vi "DataViewer.vi"() -> ()   [LabVIEW 2013]
uses:
  <vilib>/Utility/file.llb/Read From Spreadsheet File (string).vi
  <vilib>/Utility/file.llb/Read From Spreadsheet File (DBL).vi
  <vilib>/Analysis/1siggen.llb/Ramp Pattern by Delta.vi
  <vilib>/regexp/Match Regular Expression.xnode
  <vilib>/Analysis/NI_AALBase.lvlib
panel:
  in  "View Ref":bool
  out "selected reference":path caption="selected path"
  out "Polar Plot 4":picture
  out "XY Graph 3":cluster{dbl[], dbl[]}(graph)
  out "Current Freq. 2":dbl
  in  "Update 3":bool
  out "Ref In Use":bool
  in  "Remove Ref":bool
  in  "Use Reference":bool
  in  "Choose Reference Measurement":bool
  out "XY Graph 2":cluster{dbl[], dbl[]}(graph)
  in  "Update 2":bool
  out "XY Graph":cluster{dbl[], dbl[]}(graph)
  out "Current Angle":dbl
  out "Current Freq.":dbl
  in  "Update":bool
  out "Polar Plot":picture
  in  "Select Angle":dbl(slide) min=0.0 max=360.0 step=1.0 scale=0.0..360.0
  in  "Select Frequency":dbl(slide) min=1700000000.0 max=2600000000.0 step=2250000.0 scale=1700000000.0..2600000000.0
  out "all rows":string[][](array[string])
  in  "Choose Measurement":string(combo)
  in  "Choose Setup":string(combo)
  in  "Choose Folder":bool
  in  "stop":bool
  out "selected path":path
  # "Without\nReference"
  # "With\nReference"
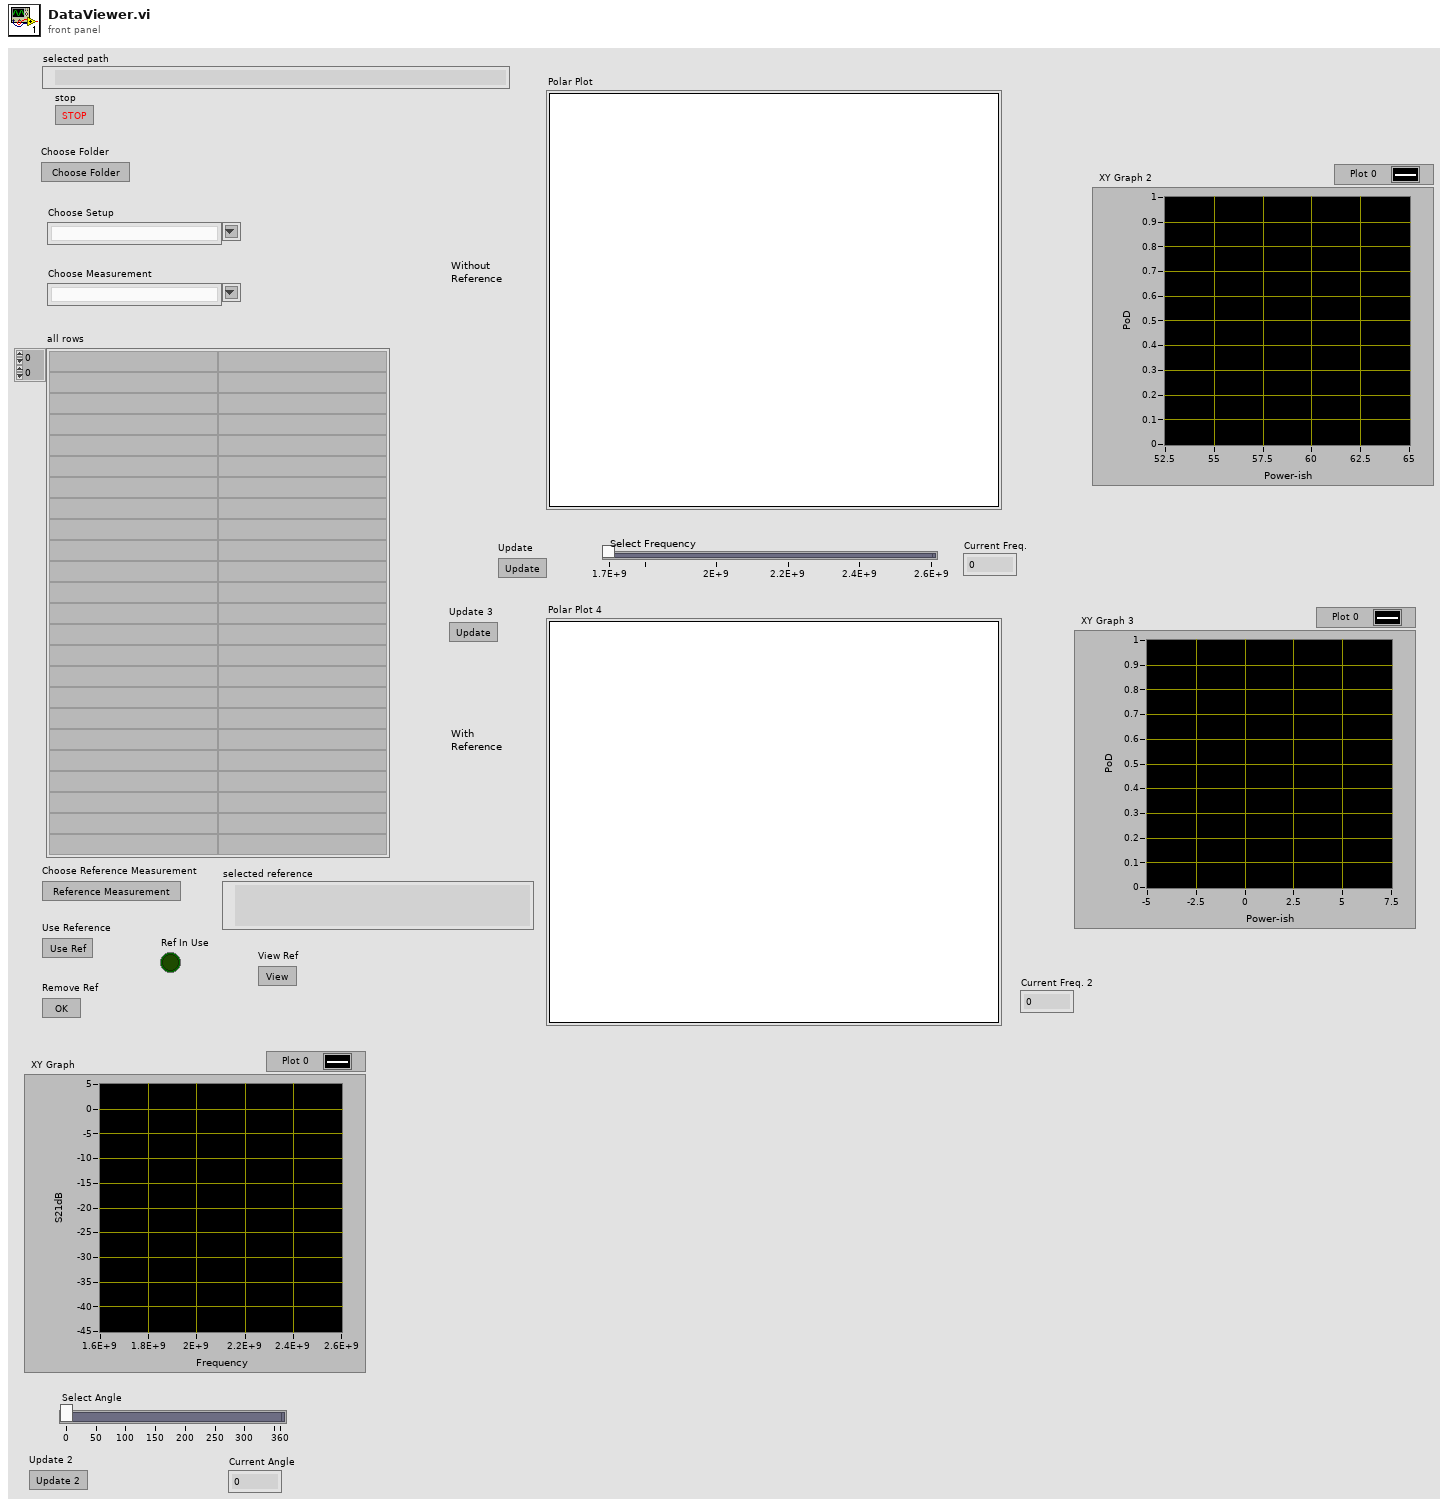
[diagram p1: front panel]
types:
  T1 = cluster{"maximum":dbl, "minimum":dbl, "clip to min":bool, "log?(F)":bool, "grid color":u32, "plot color":u32, "fmt and prec":cluster{"format":enum8{"Decimal", "Scientific", "Engineering", "Binary", "Octal", "Hex"}, "precision":u8}, "visible section":u16}
  T2 = typedef "LVBoundsTypeDef.ctl" = cluster{"Width":u32, "Height":u32}
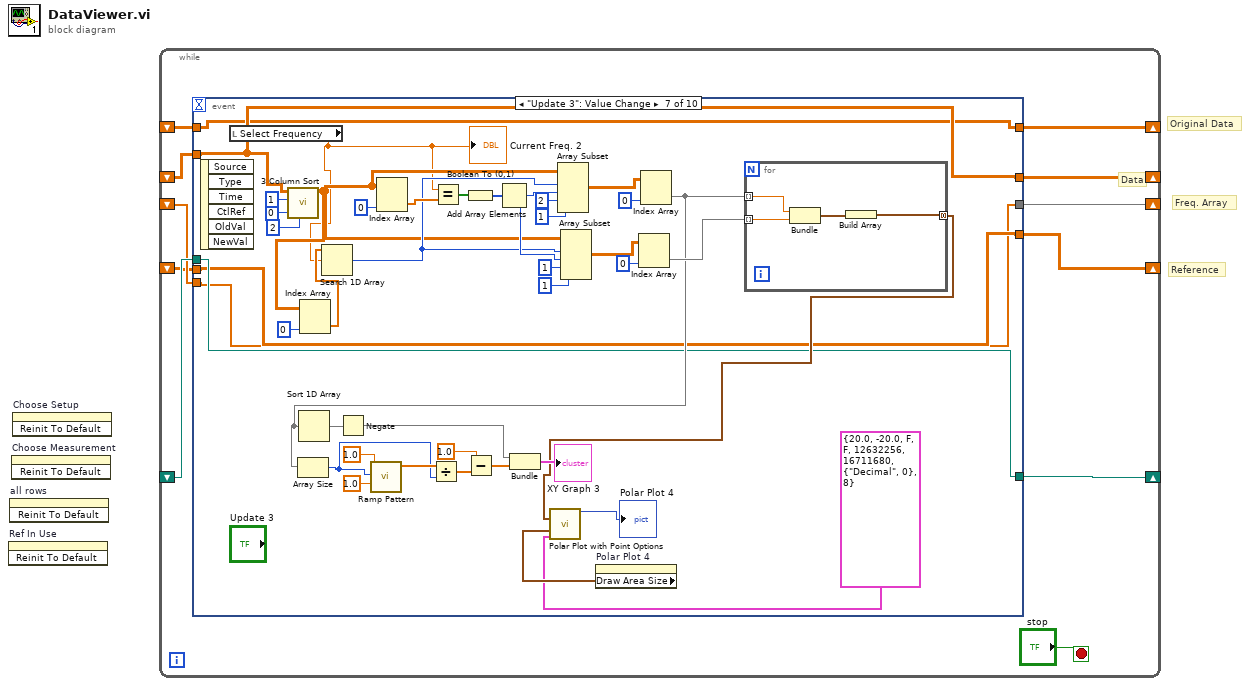
[diagram p0: block diagram]
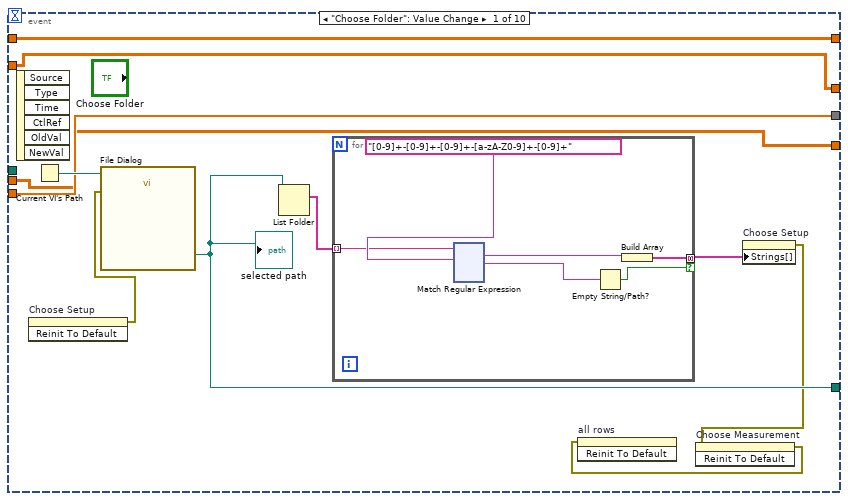
[diagram p2: hidden frame]
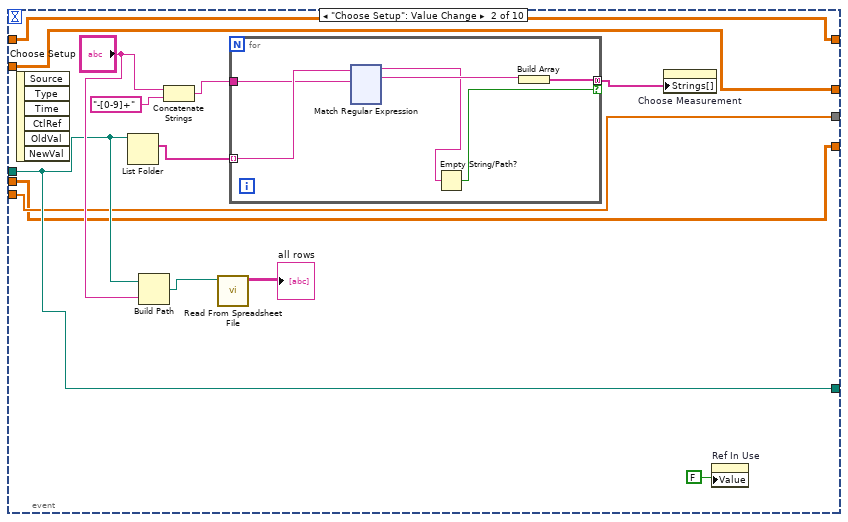
[diagram p3: hidden frame]
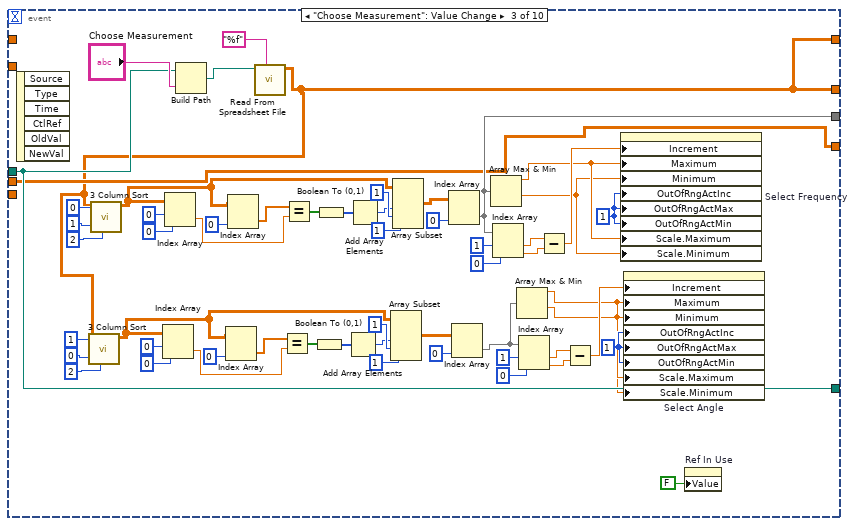
[diagram p4: hidden frame]
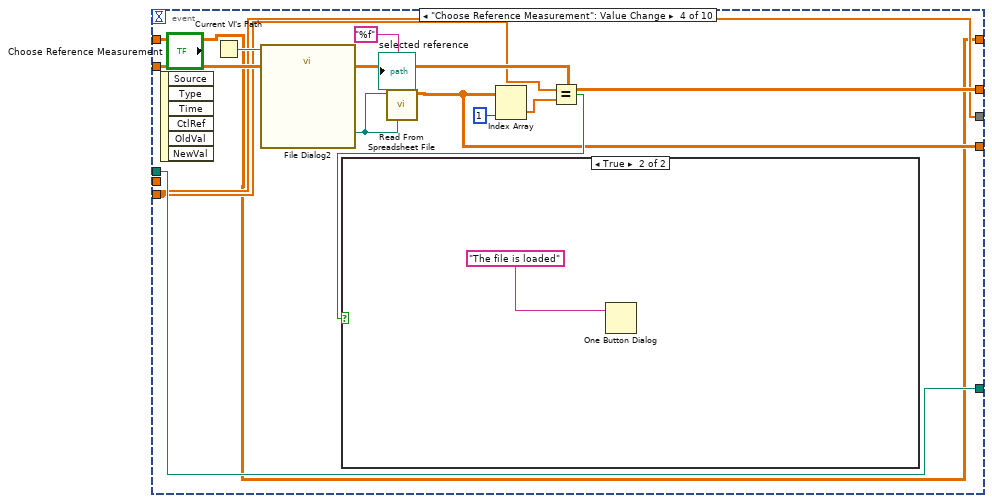
[diagram p5: hidden frame]
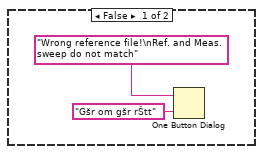
[diagram p6: hidden frame]
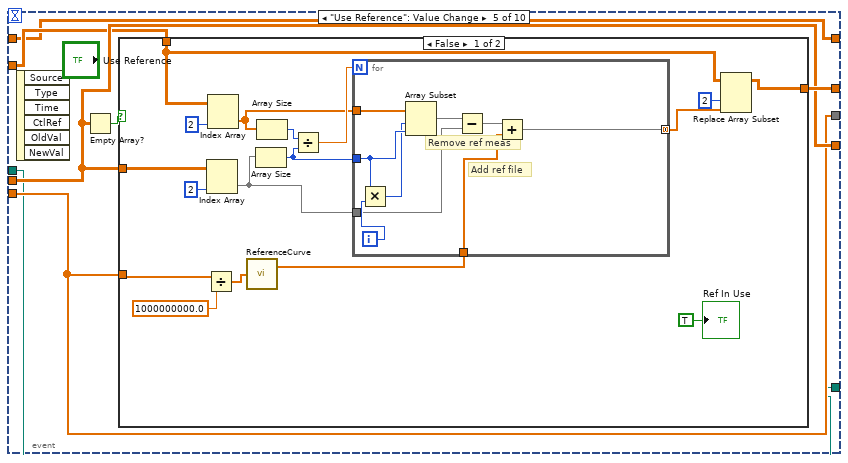
[diagram p7: hidden frame]
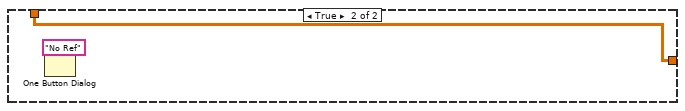
[diagram p8: hidden frame]
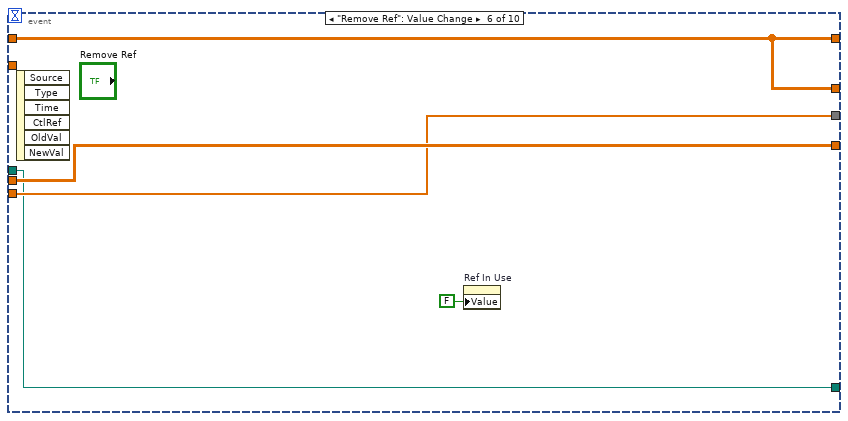
[diagram p9: hidden frame]
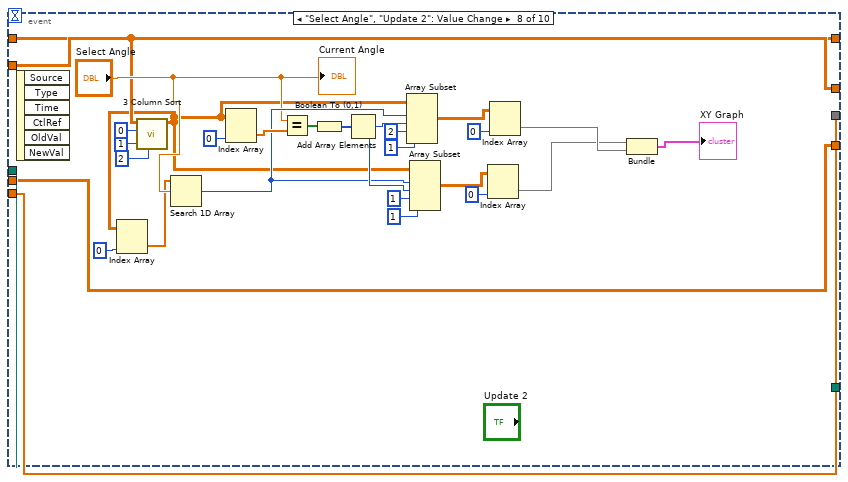
[diagram p10: hidden frame]
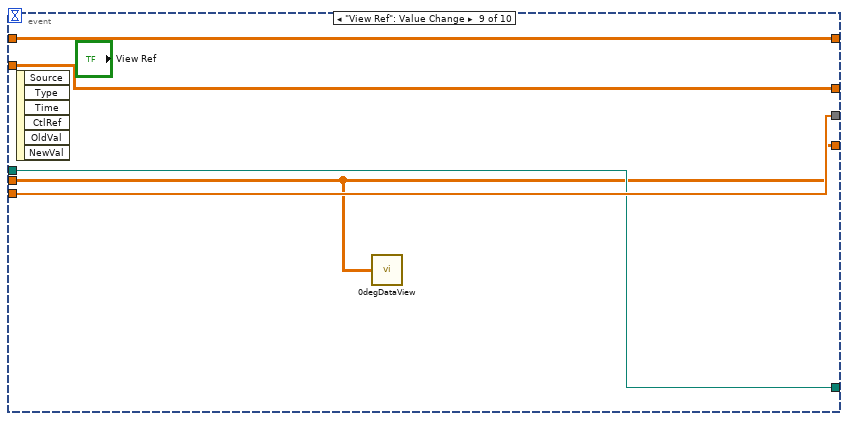
[diagram p11: hidden frame]
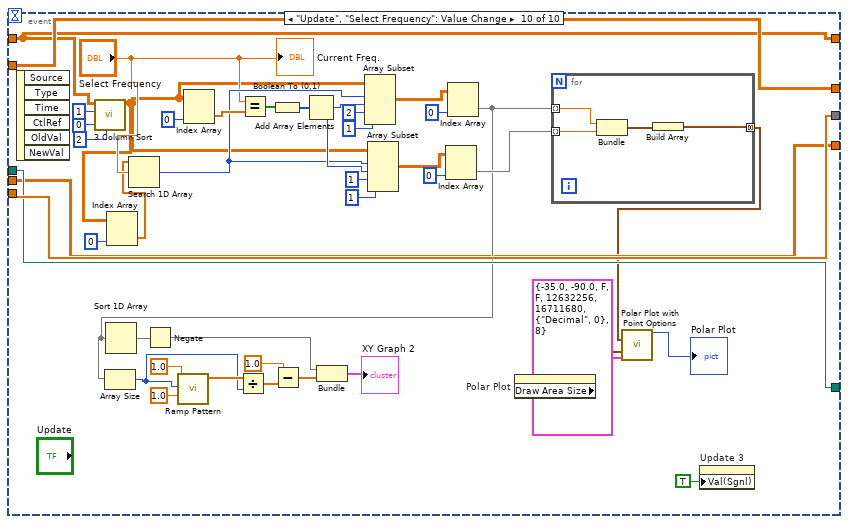
[diagram p12: hidden frame]
diagram:
  # "Reference"
  # "Original Data"
  # "Freq. Array"
  # "Data"
  n1 = invoke on="Ref In Use" class="Bool (strict)" method="Reinit To Default"() -> ()  [unwired: 3 in, 3 out]
  n2 = invoke on="all rows" class="Arr (strict)" method="Reinit To Default"() -> ()  [unwired: 3 in, 3 out]
  n3 = invoke on="Choose Measurement" class="CmbBox" method="Reinit To Default"() -> ()  [unwired: 3 in, 3 out]
  n4 = invoke on="Choose Setup" class="CmbBox" method="Reinit To Default"() -> ()  [unwired: 3 in, 3 out]
  n5 = while {
    shift-right: [w10] -> _
    shift-left: _ -> [w9]
    shift-right: [w8] -> _
    shift-left: _ -> [w3]
    shift-right: [w7] -> _
    shift-left: _ -> [w6]
    shift-right: [w5] -> _
    shift-left: _ -> [w4]
    shift-right: [w2] -> _
    shift-left: _ -> [w1]
    stop <- "stop" stop-if-true
    n6 = event shown="[6] \"Update 3\": Value Change" {
      selector: _ -> [_ _ _ _ _ _ _ _ _ _]
      dyn-events: _ -> [_ _ _ _ _ _ _ _ _ _]
      timeout: _ -> [_ _ _ _ _ _ _ _ _ _]
      tunnel: [w20 w149 w330 w336 w348 w383 w393 w460 w463 w487] -> w10
      tunnel: w9 -> [_ w149 w330 w336 w348 w383 w393 w460 w463 w487]
      tunnel: [w15 w147 w277 w335 w352 w382 w390 w441 w465 w491] -> w8
      tunnel: w3 -> [w15 w147 _ w335 w349 _ w390 w441 w465 w491]
      tunnel: [w14 w146 w284 w334 w350 w385 w391 w461 w464 w490] -> w7
      tunnel: w6 -> [w14 w146 _ w334 w350 w385 w391 w461 w464 w490]
      tunnel: [w13 w145 w278 w337 w351 w386 w392 w434 w462 w470] -> w5
      tunnel: w4 -> [w13 w145 w278 _ w351 w386 w392 w434 w462 w470]
      tunnel: [w12 w144 w277 w333 w347 w382 w389 w433 w466 w468] -> w2
      tunnel: w1 -> [w12 w144 _ w333 w347 w382 w389 w433 w466 w468]
      event "Choose Folder": Value Change {
        n7 = event-data() -> ()  [unwired: 1 in, 6 out]
        n8 = invoke on="Choose Setup" class="CmbBox" method="Reinit To Default"() -> (error out=w18:errorcluster)  [unwired: 3 in, 2 out]
        n9 = Current VI's Path() -> (path=w22:path)
        n10 = call "File Dialog"("start path"=w22, "error in"=w18) -> ("selected path"=w20:path)  [unwired: 10 in, 3 out]
        "selected path" <- w20
        n11 = List Folder(path=w20) -> (filenames=w21:string[])  [unwired: 3 in, 3 out]
        n12 = for {
          tunnel: w21 -> [w27] mode=indexing
          tunnel: [w25] -> w19 mode=concatenating if=w23
          n13 = xnode "Match Regular Expression"("input string"=w27, "regular expression"="[0-9]+-[0-9]+-[0-9]+-[a-zA-Z0-9]+-[0-9]+") -> ("whole match"=w26:string, "after match"=w24:string)  [unwired: 4 in, 3 out]
          n14 = Empty String/Path?(string/path=w24) -> (empty?=w23:bool)
          n15 = Build Array(w26) -> (w25:string[])
        }
        n16 = property on="Choose Setup" class="CmbBox"("Strings[]"=w19) -> (error out=w17:errorcluster)  [unwired: 2 in, 1 out]
        n17 = invoke on="Choose Measurement" class="CmbBox" method="Reinit To Default"(error in=w17) -> (error out=w16:errorcluster)  [unwired: 2 in, 2 out]
        n18 = invoke on="all rows" class="Arr (strict)" method="Reinit To Default"(error in=w16) -> ()  [unwired: 2 in, 3 out]
      }
      event "Choose Setup": Value Change {
        n19 = event-data() -> ()  [unwired: 1 in, 6 out]
        n20 = List Folder(path=w149) -> (filenames=w155:string[])  [unwired: 3 in, 3 out]
        n21 = Build Path(base path=w149, name or relative path="Choose Setup") -> (appended path=w148:path)
        n22 = Concatenate Strings("Choose Setup", "-[0-9]+") -> (w153:string)
        n23 = call-poly <vilib>:"Read From Spreadsheet File.vi"("file path (dialog if empty)"=w148) -> ("all rows"=→"all rows":string[][])  [unwired: 6 in, 4 out]
        n24 = for {
          tunnel: w155 -> [w161] mode=indexing
          tunnel: [w159] -> w151 mode=concatenating if=w158
          tunnel: w153 -> [w157]
          n25 = xnode "Match Regular Expression"("input string"=w161, "regular expression"=w157) -> ("before match"=w156:string, "whole match"=w160:string)  [unwired: 4 in, 3 out]
          n26 = Empty String/Path?(string/path=w156) -> (empty?=w158:bool)
          n27 = Build Array(w160) -> (w159:string[])
        }
        n28 = property on="Choose Measurement" class="CmbBox"("Strings[]"=w151) -> ()  [unwired: 2 in, 2 out]
        n29 = property on="Ref In Use" class="Bool (strict)"("Value"=FALSE ("Ref In Use")) -> ()  [unwired: 2 in, 2 out]
      }
      event "Choose Measurement": Value Change {
        w285 = u8 1 ("Response to Value Outside Limits:Maximum")
        w287 = u8 1 ("Response to Value Outside Limits:Maximum")
        n30 = event-data() -> ()  [unwired: 1 in, 6 out]
        n31 = Build Path(base path=w330, name or relative path="Choose Measurement") -> (appended path=w332:path)
        n32 = call-poly <vilib>:"Read From Spreadsheet File.vi"("format (%.3f)"="%f" ("format (%s)"), "file path (dialog if empty)"=w332) -> ("all rows"=w277:dbl[][])  [unwired: 5 in, 4 out]
        n33 = call "3 Column Sort.vi"("Tertiary Column"=2 ("index (col)"), "Secondary Column"=0 ("index (col)"), "Primary Column"=1 ("disabled index (col)"), "3 Column Array"=w277) -> ("Sorted Array"=w304:dbl[][])  [unwired: 7 in]
        n34 = call "3 Column Sort.vi"("Tertiary Column"=2 ("index (col)"), "Secondary Column"=1 ("index (col)"), "Primary Column"=0 ("disabled index (col)"), "3 Column Array"=w277) -> ("Sorted Array"=w318:dbl[][])  [unwired: 7 in]
        n35 = Index Array(array=w304, index (row)=0, index (col)=0 ("disabled index (col)")) -> (element=w311:dbl)
        n36 = Index Array(array=w318, index (row)=0, index (col)=0 ("disabled index (col)")) -> (element=w325:dbl)
        n37 = Index Array(array=w304, index (col)=0 ("disabled index (col)")) -> (element=w312:dbl[])  [unwired: 1 in]
        n38 = Index Array(array=w318, index (col)=0 ("disabled index (col)")) -> (element=w326:dbl[])  [unwired: 1 in]
        n39 = Equal?(x=w312, y=w311) -> (x = y?=w310:bool[])
        n40 = Equal?(x=w326, y=w325) -> (x = y?=w324:bool[])
        n41 = Boolean To (0,1)(Boolean=w310) -> (0, 1=w305:i16[])
        n42 = Boolean To (0,1)(Boolean=w324) -> (0, 1=w319:i16[])
        n43 = Add Array Elements(numeric array=w305) -> (sum=w302:i16)
        n44 = Add Array Elements(numeric array=w319) -> (sum=w316:i16)
        n45 = Array Subset(array=w304, length (row)=w302, index (col)=1 ("index"), length (col)=1 ("length")) -> (w297:dbl[][])  [unwired: 1 in]
        n46 = Array Subset(array=w318, length (row)=w316, index (col)=1 ("index"), length (col)=1 ("length")) -> (w300:dbl[][])  [unwired: 1 in]
        n47 = Index Array(array=w300, index (col)=0 ("disabled index (col)")) -> (element=w284:dbl[])  [unwired: 1 in]
        n48 = Index Array(array=w297, index (col)=0 ("disabled index (col)")) -> (element=w281:dbl[])  [unwired: 1 in]
        n49 = Array Max & Min(array=w284) -> (max value=w283:dbl, min value=w282:dbl)  [unwired: 2 out]
        n50 = Index Array(array=w284, index #1=1 ("index"), index #2=0 ("index")) -> (element #1=w294:dbl, element #2=w293:dbl)
        n51 = Array Max & Min(array=w281) -> (max value=w280:dbl, min value=w279:dbl)  [unwired: 2 out]
        n52 = Index Array(array=w281, index #1=1 ("index"), index #2=0 ("index")) -> (element #1=w290:dbl, element #2=w289:dbl)
        n53 = Subtract(x=w294, y=w293) -> (x-y=w286:dbl)
        n54 = Subtract(x=w290, y=w289) -> (x-y=w288:dbl)
        n55 = property on="Select Frequency" class="Slide (strict)"("Increment"=w286, "Maximum"=w283, "Minimum"=w282, "OutOfRngActInc"=w285, "OutOfRngActMax"=w285, "OutOfRngActMin"=w285, "Scale.Maximum"=w283, "Scale.Minimum"=w282) -> ()  [unwired: 2 in, 2 out]
        n56 = property on="Select Angle" class="Slide (strict)"("Increment"=w288, "Maximum"=w280, "Minimum"=w279, "OutOfRngActInc"=w287, "OutOfRngActMax"=w287, "OutOfRngActMin"=w287, "Scale.Maximum"=w280, "Scale.Minimum"=w279) -> ()  [unwired: 2 in, 2 out]
        n57 = property on="Ref In Use" class="Bool (strict)"("Value"=FALSE ("Ref In Use")) -> ()  [unwired: 2 in, 2 out]
      }
      event "Choose Reference Measurement": Value Change {
        n58 = event-data() -> ()  [unwired: 1 in, 6 out]
        n59 = Current VI's Path() -> (path=w343:path)
        n60 = call "File Dialog2"("start path"=w343) -> ("selected path"=w341:path)  [unwired: 11 in, 3 out]
        "selected reference" <- w341
        n61 = call-poly <vilib>:"Read From Spreadsheet File.vi"("format (%.3f)"="%f" ("format (%s)"), "file path (dialog if empty)"=w341) -> ("all rows"=w337:dbl[][])  [unwired: 5 in, 4 out]
        n62 = Index Array(array=w337, index (col)=1 ("disabled index (col)")) -> (element=w339:dbl[])  [unwired: 1 in]
        n63 = Equal?(x=w334, y=w339) -> (x = y?=w338:bool)
        n64 = case shown="True" w338 {
          frame False {
            n65 = One Button Dialog(message="Wrong reference file!\nRef. and Meas. sweep do not match", button name ("OK")="Gšr om gšr rŠtt") -> ()  [unwired: 1 out]
          }
          frame True {
            n66 = One Button Dialog(message="The file is loaded") -> ()  [unwired: 1 in, 1 out]
          }
        }
      }
      event "Use Reference": Value Change {
        n67 = event-data() -> ()  [unwired: 1 in, 6 out]
        n68 = Empty Array?(array=w351) -> (empty?=w353:bool)
        n69 = case shown="False" w353 {
          tunnel: w351 -> [w369 _]
          tunnel: w350 -> [w362 _]
          tunnel: [w355 w380] -> w352
          tunnel: w349 -> [w358 w380]
          frame False {
            n70 = Divide(x=w362, y=1000000000.0) -> (x/y=w363:dbl[])
            n71 = Index Array(array=w369, index (col)=2 ("disabled index (col)")) -> (element=w364:dbl[])  [unwired: 1 in]
            n72 = Index Array(array=w358, index (col)=2 ("disabled index (col)")) -> (element=w359:dbl[])  [unwired: 1 in]
            n73 = call "ReferenceCurve.vi"("Frequency(GHz)"=w363) -> ("SGH Gain"=w354:dbl[])  [unwired: 1 out]
            n74 = Array Size(array=w364) -> (size(s)=w365:i32)
            n75 = Array Size(array=w359) -> (size(s)=w367:i32)
            n76 = Divide(x=w367, y=w365) -> (x/y=w366:dbl)
            n77 = for {
              N: w366 -> [_]
              tunnel: w365 -> [w378]
              tunnel: w364 -> [w376]
              tunnel: w354 -> [w374]
              tunnel: [w373] -> w357 mode=concatenating
              tunnel: w359 -> [w372]
              i -> [w379]
              # "Remove ref meas"
              # "Add ref file"
              n78 = Multiply(x=w378, y=w379) -> (x*y=w377:i32)
              n79 = Array Subset(array=w372, index=w377, length=w378) -> (w371:dbl[])
              n80 = Subtract(x=w371, y=w376) -> (x-y=w375:dbl[])
              n81 = Add(x=w375, y=w374) -> (x+y=w373:dbl[])
            }
            n82 = Replace Array Subset(array=w358, new element=w357, index (col)=2 ("disabled index (col)")) -> (w355:dbl[][])  [unwired: 1 in]
            "Ref In Use" <- TRUE ("Ref In Use")
          }
          frame True {
            n83 = One Button Dialog(message="No Ref") -> ()  [unwired: 1 in, 1 out]
          }
        }
      }
      event "Remove Ref": Value Change {
        n84 = event-data() -> ()  [unwired: 1 in, 6 out]
        n85 = property on="Ref In Use" class="Bool (strict)"("Value"=FALSE ("Ref In Use")) -> ()  [unwired: 2 in, 2 out]
      }
      event "Update 3": Value Change {
        n86 = event-data() -> ()  [unwired: 1 in, 6 out]
        n87 = local read "Select Frequency"() -> (w388:dbl)
        "Current Freq. 2" <- w388
        n88 = call "3 Column Sort.vi"("Tertiary Column"=2, "Secondary Column"=0, "Primary Column"=1, "3 Column Array"=w390) -> ("Sorted Array"=w409:dbl[][])  [unwired: 7 in]
        n89 = Index Array(array=w409, index (col)=0 ("disabled index (col)")) -> (element=w408:dbl[])  [unwired: 1 in]
        n90 = Search 1D Array(1D array=w408, element=w388) -> (index of element=w416:i32)  [unwired: 1 in]
        n91 = Index Array(array=w409, index (col)=0 ("disabled index (col)")) -> (element=w426:dbl[])  [unwired: 1 in]
        n92 = Equal?(x=w388, y=w426) -> (x = y?=w425:bool[])
        n93 = Boolean To (0,1)(Boolean=w425) -> (0, 1=w428:i16[])
        n94 = Add Array Elements(numeric array=w428) -> (sum=w417:i16)
        n95 = Array Subset(array=w409, index (row)=w416, length (row)=w417, index (col)=2 ("index"), length (col)=1 ("length")) -> (w415:dbl[][])
        n96 = Array Subset(array=w409, index (row)=w416, length (row)=w417, index (col)=1 ("index"), length (col)=1 ("length")) -> (w414:dbl[][])
        n97 = property on="Polar Plot 4" class="Pict"() -> ("Draw Area Size"=w396:T2)  [unwired: 2 in, 2 out]
        n98 = Index Array(array=w414, index (col)=0 ("disabled index (col)")) -> (element=w413:dbl[])  [unwired: 1 in]
        n99 = Index Array(array=w415, index (col)=0 ("disabled index (col)")) -> (element=w406:dbl[])  [unwired: 1 in]
        n100 = Array Size(array=w406) -> (size(s)=w402:i32)
        n101 = Sort 1D Array(array=w406) -> (sorted array=w407:dbl[])
        n102 = Negate(x=w407) -> (-x=w398:dbl[])
        n103 = call-poly <vilib>:"Ramp Pattern.vi"("start"=1.0, "end"=w402, "delta"=1.0) -> ("Ramp Pattern"=w403:dbl[])  [unwired: 6 in, 2 out]
        n104 = Divide(x=w403, y=w402) -> (x/y=w400:dbl[])
        n105 = Subtract(x=1.0, y=w400) -> (x-y=w399:dbl[])
        n106 = Bundle(w398, w399) -> (→"XY Graph 3":cluster{dbl[], dbl[]})  [unwired: 1 in]
        n107 = for {
          tunnel: w406 -> [w432] mode=indexing
          tunnel: w413 -> [w431] mode=indexing
          tunnel: [w429] -> w394 mode=concatenating
          n108 = Bundle(w432, w431) -> (w430:cluster{dbl, dbl})  [unwired: 1 in]
          n109 = Build Array(w430) -> (w429:cluster{dbl, dbl}[])
        }
        n110 = call <vilib>:"Polar Plot with Point Options.vi"("data array [mag, phase (deg)]"=w394, "dimensions (w,h)"=w396, "polar attributes"=T1 {"maximum"=20.0, "minimum"=-20.0, "clip to min"=FALSE, "log?(F)"=FALSE, "grid color"=12632256, "plot color"=16711680, "fmt and prec"={"format"=enum."Decimal", "precision"=0}, "visible section"=8}) -> ("new picture"=→"Polar Plot 4":picture)  [unwired: 12 in]
      }
      event "Select Angle", "Update 2": Value Change {
        n111 = event-data() -> ()  [unwired: 1 in, 6 out]
        n112 = call "3 Column Sort.vi"("Tertiary Column"=2, "Secondary Column"=1, "Primary Column"=0, "3 Column Array"=w441) -> ("Sorted Array"=w436:dbl[][])  [unwired: 7 in]
        n113 = Index Array(array=w436, index (col)=0 ("disabled index (col)")) -> (element=w435:dbl[])  [unwired: 1 in]
        n114 = Search 1D Array(1D array=w435, element="Select Angle") -> (index of element=w447:i32)  [unwired: 1 in]
        n115 = Index Array(array=w436, index (col)=0 ("disabled index (col)")) -> (element=w457:dbl[])  [unwired: 1 in]
        n116 = Equal?(x="Select Angle", y=w457) -> (x = y?=w456:bool[])
        n117 = Boolean To (0,1)(Boolean=w456) -> (0, 1=w459:i16[])
        n118 = Add Array Elements(numeric array=w459) -> (sum=w448:i16)
        n119 = Array Subset(array=w436, index (row)=w447, length (row)=w448, index (col)=2 ("index"), length (col)=1 ("length")) -> (w446:dbl[][])
        n120 = Array Subset(array=w436, index (row)=w447, length (row)=w448, index (col)=1 ("index"), length (col)=1 ("length")) -> (w445:dbl[][])
        n121 = Index Array(array=w445, index (col)=0 ("disabled index (col)")) -> (element=w438:dbl[])  [unwired: 1 in]
        n122 = Index Array(array=w446, index (col)=0 ("disabled index (col)")) -> (element=w439:dbl[])  [unwired: 1 in]
        n123 = Bundle(w438, w439) -> (→"XY Graph":cluster{dbl[], dbl[]})  [unwired: 1 in]
        "Current Angle" <- "Select Angle"
      }
      event "View Ref": Value Change {
        n124 = event-data() -> ()  [unwired: 1 in, 6 out]
        n125 = call "0degDataView.vi"("3 Column Array"=w462) -> ()
      }
      event "Update", "Select Frequency": Value Change {
        n126 = event-data() -> ()  [unwired: 1 in, 6 out]
        n127 = call "3 Column Sort.vi"("Tertiary Column"=2, "Secondary Column"=0, "Primary Column"=1, "3 Column Array"=w468) -> ("Sorted Array"=w484:dbl[][])  [unwired: 7 in]
        n128 = Index Array(array=w484, index (col)=0 ("disabled index (col)")) -> (element=w483:dbl[])  [unwired: 1 in]
        n129 = Search 1D Array(1D array=w483, element="Select Frequency") -> (index of element=w495:i32)  [unwired: 1 in]
        n130 = Index Array(array=w484, index (col)=0 ("disabled index (col)")) -> (element=w505:dbl[])  [unwired: 1 in]
        n131 = Equal?(x="Select Frequency", y=w505) -> (x = y?=w504:bool[])
        n132 = Boolean To (0,1)(Boolean=w504) -> (0, 1=w507:i16[])
        n133 = Add Array Elements(numeric array=w507) -> (sum=w496:i16)
        n134 = Array Subset(array=w484, index (row)=w495, length (row)=w496, index (col)=2 ("index"), length (col)=1 ("length")) -> (w494:dbl[][])
        n135 = Array Subset(array=w484, index (row)=w495, length (row)=w496, index (col)=1 ("index"), length (col)=1 ("length")) -> (w493:dbl[][])
        n136 = Index Array(array=w493, index (col)=0 ("disabled index (col)")) -> (element=w492:dbl[])  [unwired: 1 in]
        n137 = Index Array(array=w494, index (col)=0 ("disabled index (col)")) -> (element=w480:dbl[])  [unwired: 1 in]
        n138 = Array Size(array=w480) -> (size(s)=w476:i32)
        n139 = Sort 1D Array(array=w480) -> (sorted array=w481:dbl[])
        n140 = Negate(x=w481) -> (-x=w472:dbl[])
        n141 = call-poly <vilib>:"Ramp Pattern.vi"("start"=1.0, "end"=w476, "delta"=1.0) -> ("Ramp Pattern"=w477:dbl[])  [unwired: 6 in, 2 out]
        n142 = Divide(x=w477, y=w476) -> (x/y=w474:dbl[])
        n143 = Subtract(x=1.0, y=w474) -> (x-y=w473:dbl[])
        n144 = Bundle(w472, w473) -> (→"XY Graph 2":cluster{dbl[], dbl[]})  [unwired: 1 in]
        n145 = property on="Polar Plot" class="Pict"() -> ("Draw Area Size"=w509:T2)  [unwired: 2 in, 2 out]
        n146 = for {
          tunnel: w480 -> [w513] mode=indexing
          tunnel: w492 -> [w512] mode=indexing
          tunnel: [w510] -> w469 mode=concatenating
          n147 = Bundle(w513, w512) -> (w511:cluster{dbl, dbl})  [unwired: 1 in]
          n148 = Build Array(w511) -> (w510:cluster{dbl, dbl}[])
        }
        n149 = call <vilib>:"Polar Plot with Point Options.vi"("data array [mag, phase (deg)]"=w469, "dimensions (w,h)"=w509, "polar attributes"=T1 {"maximum"=-35.0, "minimum"=-90.0, "clip to min"=FALSE, "log?(F)"=FALSE, "grid color"=12632256, "plot color"=16711680, "fmt and prec"={"format"=enum."Decimal", "precision"=0}, "visible section"=8}) -> ("new picture"=→"Polar Plot":picture)  [unwired: 12 in]
        n150 = property on="Update 3" class="Bool (strict)"("Val(Sgnl)"=TRUE ("Value (Signaling)")) -> ()  [unwired: 2 in, 2 out]
        "Current Freq." <- "Select Frequency"
      }
    }
  }
